vi "subXMLGetAllValuesFromSection.vi"(8 "error in (no error)":errorcluster, 10 "XPath expression":string, 11 "Refnum in":refnum<k20>) -> (0 "error out":errorcluster, 1 "Values":string[](array[string]), 3 "Refnum out":refnum<k20>)   [LabVIEW 2019, in "SolutionBuilder.lvlib" / "SolutionBuilder.lvclass"]
uses:
  SolutionBuilder.lvclass
  <vilib>/xml/NI_XML.lvlib
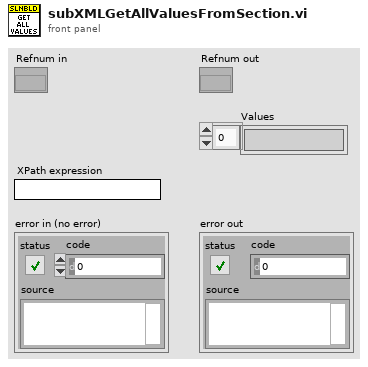
[diagram p1: front panel]
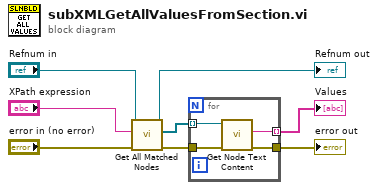
[diagram p0: block diagram]
diagram:
  n1 = call <vilib>:"Get All Matched Nodes.vi"("error in (no error)"="error in (no error)", "XPath expression"="XPath expression", "node in"="Refnum in") -> ("error out"=w2:errorcluster, "node result array"=w3:refnum<k20>[], "node out"=→"Refnum out":refnum<k20>)  [unwired: 6 in]
  n2 = for {
    tunnel: w2 -> [w12]
    tunnel: w3 -> [w11] mode=indexing
    tunnel: [w9] -> w8 mode=indexing
    tunnel: [w10] -> w6
    n3 = call <vilib>:"Get Node Text Content.vi"("error in (no error)"=w12, "node in"=w11) -> ("error out"=w10:errorcluster, "node text"=w9:string)  [unwired: 7 in, 1 out]
  }
  "Values" <- w8
  "error out" <- w6
